vi "_CSM Module Switcher.vi"() -> ()   [LabVIEW 2017]
uses:
  _Support/Typedef/_CSM_GlobalLog_MSG.ctl
  _Support/Typedef/_CSM_Response Source Message.ctl
  _Support/Typedef/_CSM_GlobalLog_MSG_TYPE.ctl
  _Support/Common/Format Timestamp.vi
  AdvanceAPI/CSM - Convert Error to Argument.vi
  <vilib>/Utility/error.llb/Clear Errors.vi
  _Support/GlobalEvent/Gevt-ThreadQueueName.vi
  AdvanceAPI/CSM - Keywords.vi
  _Support/Common/Trim Single line Text.vi
  AdvanceAPI/CSM - Make String Arguments Safe.vi
  _Support/GlobalEvent/FGV-GlobalEventRef.vi
  _Support/FGV-BroadcastRegistry/global-CSMQ FGV Change Flag.vi
  _Support/CSMQ/_CSMOFGV.vi
  Communicable State Machine.lvlib
  _Support/csm-tool-support.lvlib
panel:
  in  "Refresh CSMs Button":bool
  in  "CSM":string(combo)
  in  "Toolbar.Open FP":bool
  in  "Toolbar.Open BD":bool
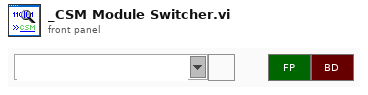
[diagram p1: front panel]
types:
  T1 = typedef "Communicable State Machine.lvlib/_CSM_GlobalLog_MSG.ctl" = cluster{"Name(\"\" to use uuid)":string, "Current State":string, "Arguments":string, "Source Message":T2, "Source Module":string, "Complete(T)/Start(F)":bool, "LogType":T3}
  T2 = typedef "Communicable State Machine.lvlib/_CSM_Response Source Message.ctl" = cluster{"‘State":string, "’Arguments":string, "’Error":errorcluster}
  T3 = typedef "Communicable State Machine.lvlib/_CSM_GlobalLog_MSG_TYPE.ctl" = enum16{"User Log", "State Change", "Status", "Interrupt", "Register", "Unregister", "Error Log", "Module Created", "Module Destroyed"}
  T4 = enum32{"Invalid", "Standard", "Closed", "Hidden", "Minimized", "Maximized"}
  T5 = enum32{"invalid app kind", "Development System", "Run Time System", "Student Edition", "Embedded LabVIEW", "Evaluation", "Custom"}
  T6 = cluster{"Shift":bool, "Ctrl":bool, "Alt":bool, "Cmd":bool, "Opt":bool}
  T7 = cluster{"Core":cluster{"Current VI Reference":refnum<vi>, "Close Panel on Exit?":bool}, "CSM Global Log Event":refnum<user-event>, "lvlps File":path, "Toobar.advance":refnum<vi>[]}
  T8 = cluster{"Current VI Reference":refnum<vi>, "Close Panel on Exit?":bool}
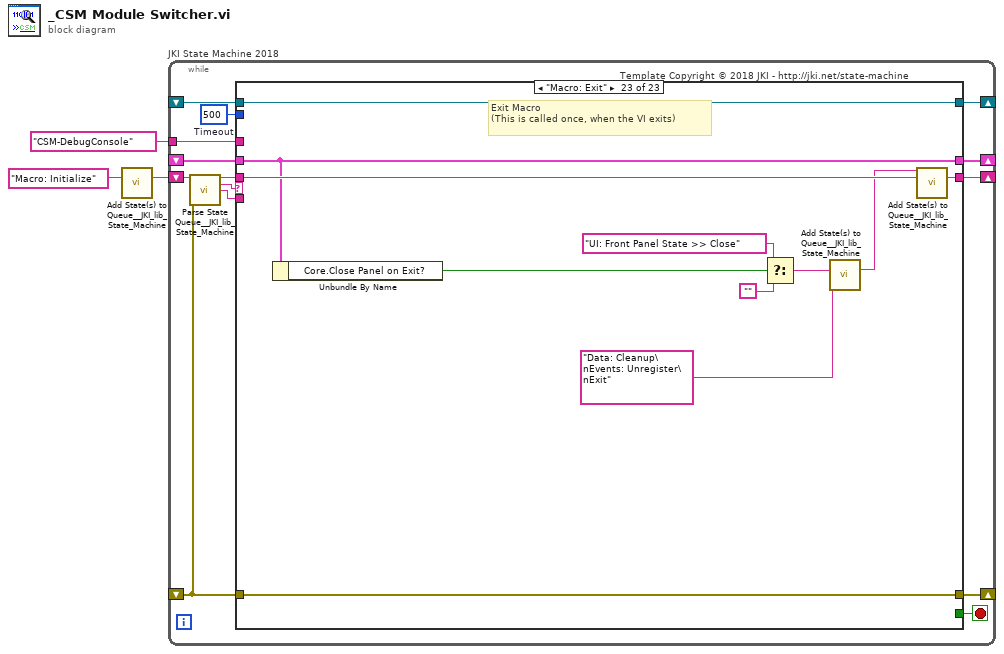
[diagram p0: block diagram]
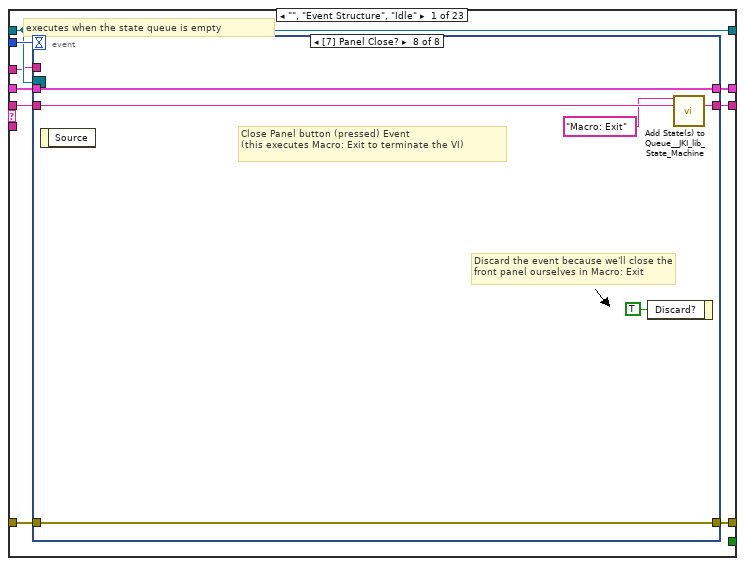
[diagram p2: hidden frame]
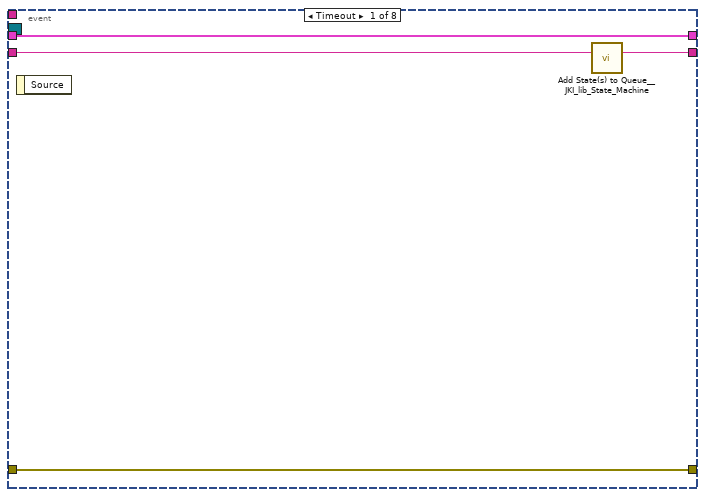
[diagram p3: hidden frame]
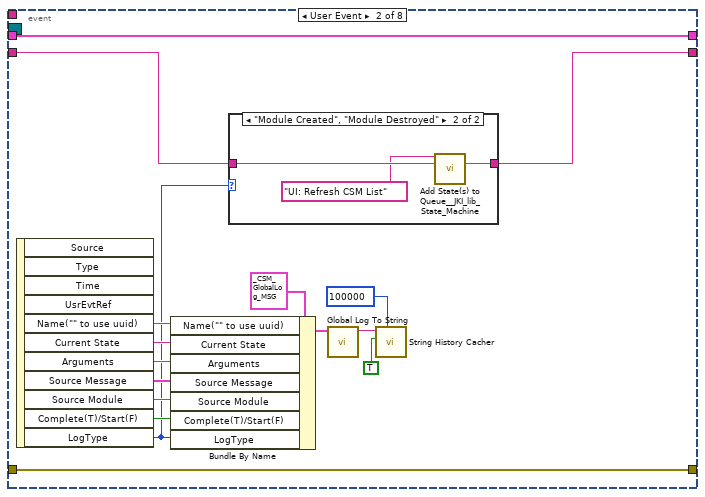
[diagram p4: hidden frame]
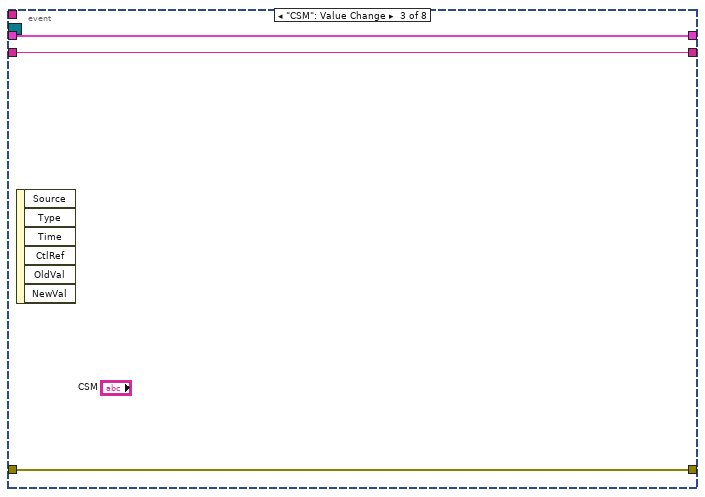
[diagram p6: hidden frame]
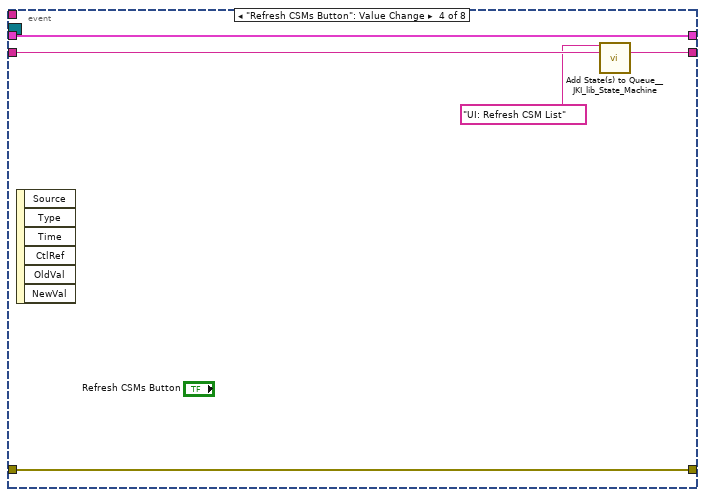
[diagram p7: hidden frame]
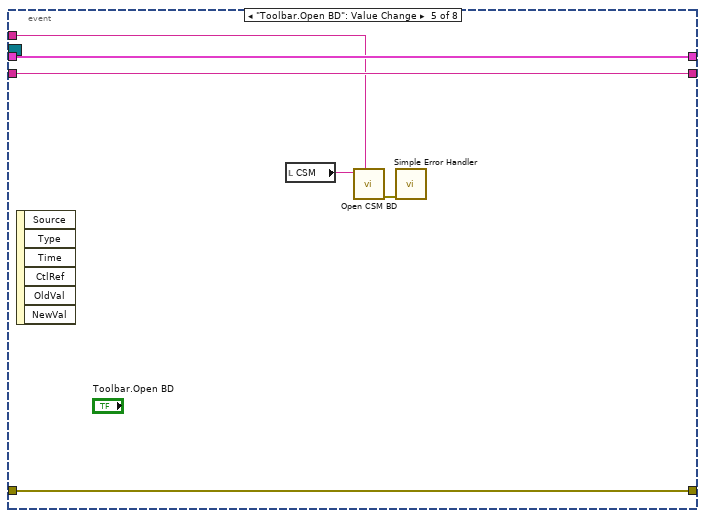
[diagram p8: hidden frame]
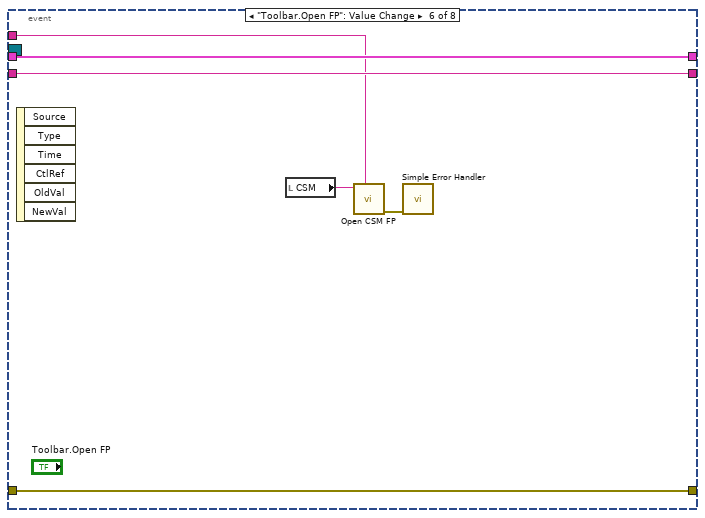
[diagram p9: hidden frame]
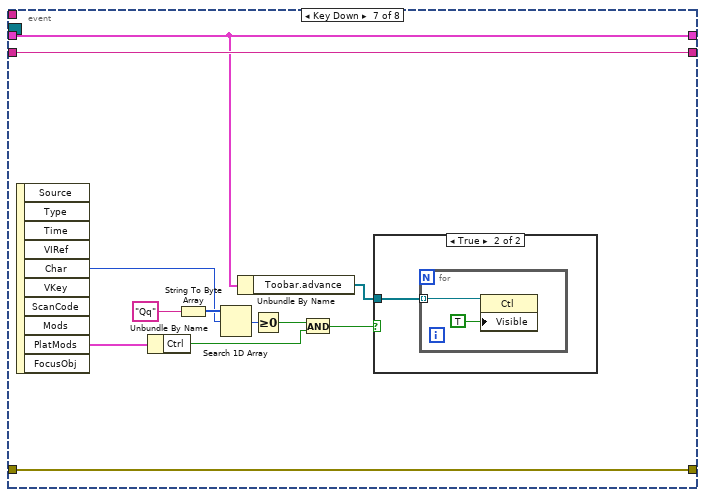
[diagram p10: hidden frame]
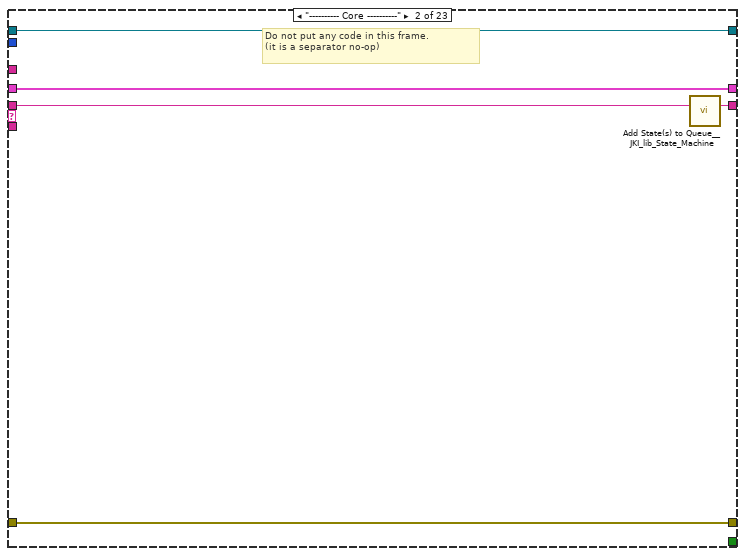
[diagram p12: hidden frame]
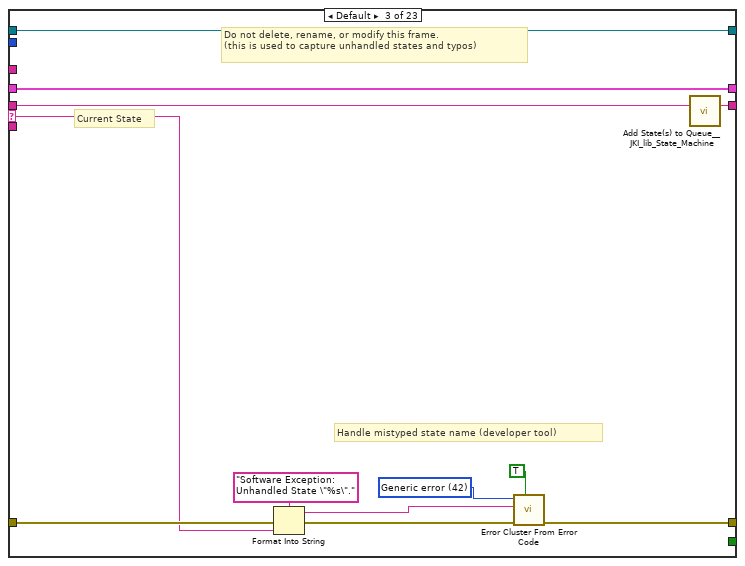
[diagram p13: hidden frame]
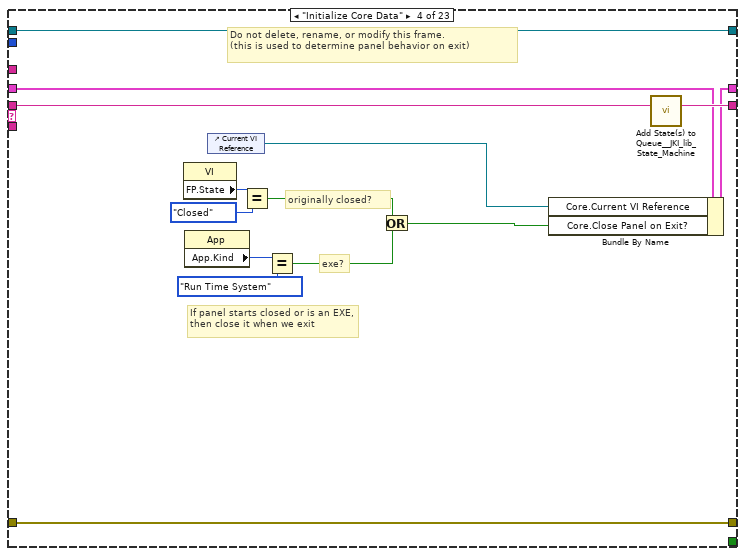
[diagram p14: hidden frame]
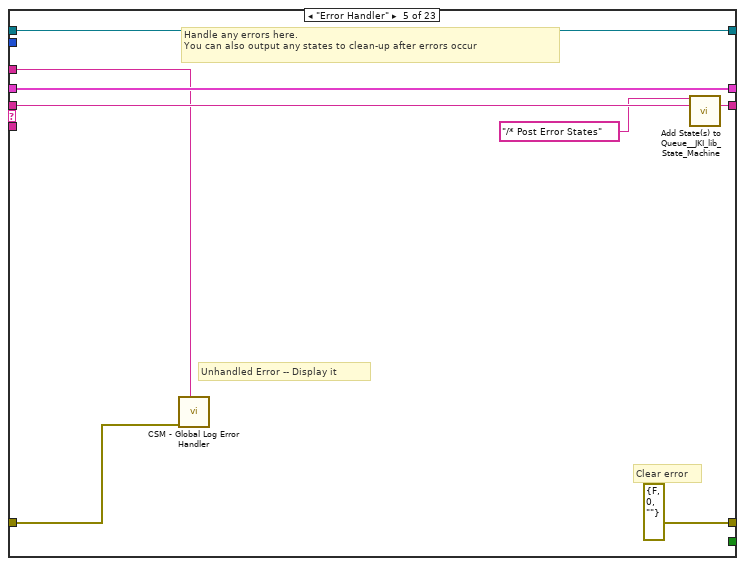
[diagram p15: hidden frame]
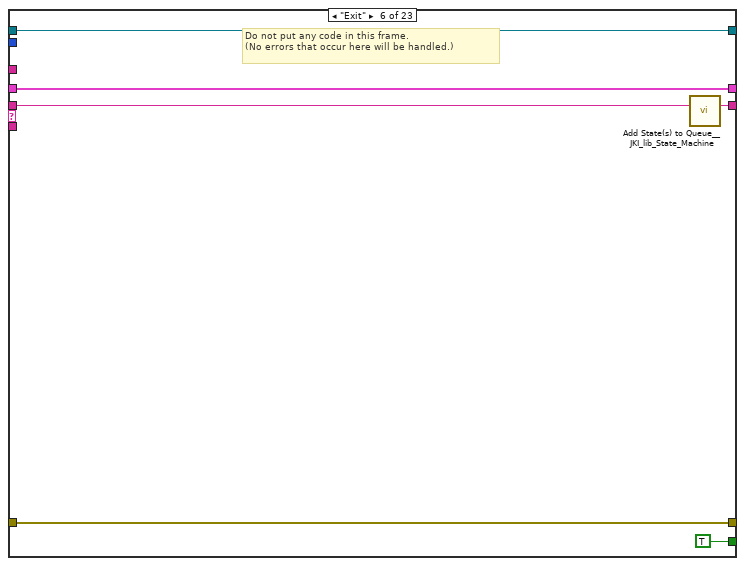
[diagram p16: hidden frame]
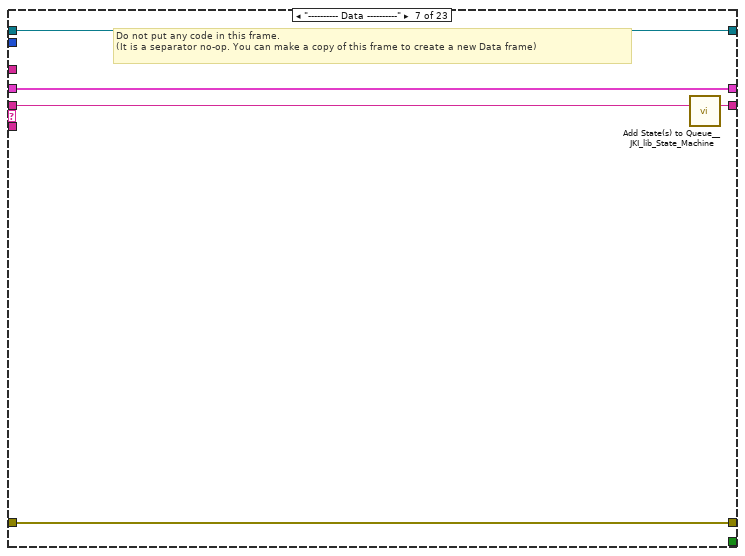
[diagram p17: hidden frame]
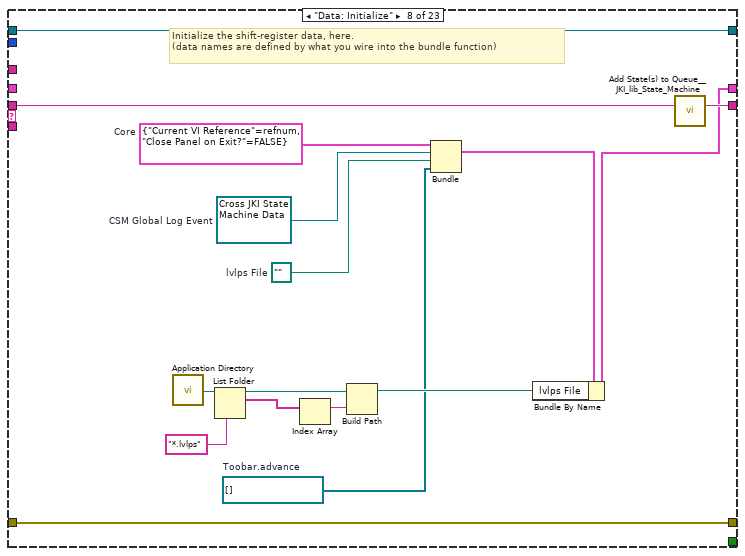
[diagram p18: hidden frame]
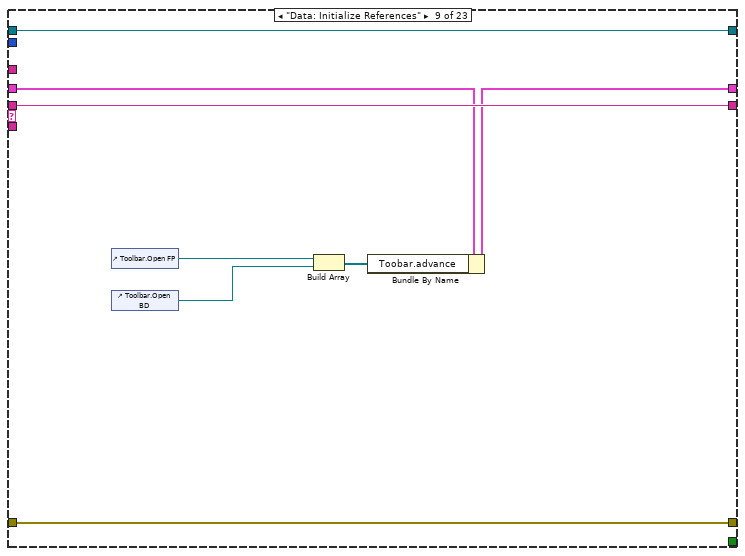
[diagram p19: hidden frame]
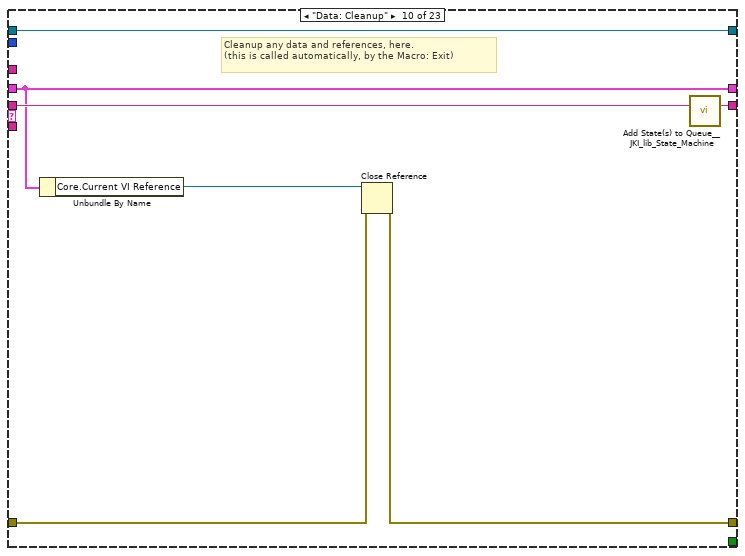
[diagram p20: hidden frame]
diagram:
  n1 = call <vilib>:"Add State(s) to Queue__JKI_lib_State_Machine.vi"("State(s) in (\"\")"="Macro: Initialize") -> ("States Out"=w2:string)  [unwired: 14 in]
  n2 = while "JKI State Machine 2018" {
    shift-right: [w10] -> _
    shift-left: _ -> [w9]
    shift-right: [w13] -> _
    shift-left: _ -> [w7]
    shift-right: [w12] -> _
    shift-left: w2 -> [w14]
    shift-right: [w6] -> _
    shift-left: _ -> [w5]
    tunnel: "CSM-DebugConsole" -> [w4]
    stop <- w11 stop-if-true
    w8 = 500  # Timeout
    # "Template Copyright © 2018 JKI - http://jki.net/state-machine"
    n3 = call <vilib>:"Parse State Queue__JKI_lib_State_Machine.vi"("State Queue"=w14, "Error In (no error)"=w7) -> ("Remaining States"=w16:string, "Current State"=w17:string, "Arguments"=w15:string)  [unwired: 11 in]
    n4 = case shown="\"Macro: Exit\"" w17 {
      selector: w17 -> [_ _ w98 _ _ _ _ _ _ _ _ _ _ _ _ _ _ _ _ _ _ _ _]
      tunnel: w16 -> [w26 w96 w102 w122 w130 w136 w141 w157 w164 w172 w177 w184 w191 w196 w202 w212 w224 w301 w316 w320 w326 w332 w343]
      tunnel: w15 -> [_ _ _ _ _ _ _ _ _ _ _ _ _ _ _ w207 w218 w299 _ _ _ _ _]
      tunnel: w9 -> [w24 w93 w100 w115 w127 w134 w138 _ w163 w167 w174 w182 w187 w193 w198 w210 w220 w296 w315 w318 w323 w329 w340]
      tunnel: [w23 w94 w104 w119 errorcluster {"status"=FALSE, "code"=0, "source"=""} ("error out") w133 w139 w154 w165 w168 w175 w180 w188 w194 w200 w208 w221 w302 w317 w321 w324 w330 w341] -> w13
      tunnel: w7 -> [w22 w94 w103 w119 w126 w133 w139 w154 w165 w169 w175 _ _ w194 w200 w209 w222 w302 w317 w321 w324 w330 w341]
      tunnel: [w25 w95 w101 w121 w129 w135 w140 w156 w164 w171 w176 w183 w190 w195 w201 w211 w223 w301 w316 w320 w325 w331 w342] -> w12
      tunnel: [_ _ _ _ _ TRUE _ _ _ _ _ _ _ _ _ _ _ _ _ _ _ _ _] -> w11
      tunnel: [w21 w93 w100 w120 w127 w134 w138 w149 w159 w167 w174 w182 w187 w193 w198 w210 w220 w296 w315 w318 w323 w329 w340] -> w10
      tunnel: w8 -> [w20 _ _ _ _ _ _ _ _ _ _ _ _ _ _ _ _ _ _ _ _ _ _]
      tunnel: [w19 w92 w97 w109 w124 w131 w137 w152 w162 w166 w173 w181 w189 w192 w199 w206 w217 w300 w314 w319 w322 w327 w333] -> w6
      tunnel: w5 -> [w19 w92 w97 w109 w124 w131 w137 w152 w162 w166 w173 _ w189 w192 w199 w206 w217 w300 w314 w319 w322 w327 w333]
      tunnel: w4 -> [w18 _ _ _ w123 _ _ _ _ _ _ _ _ _ _ _ _ _ _ _ _ _ _]
      frame "", "Event Structure", "Idle" {
        # "executes when the state queue is empty"
        n5 = event shown="[7] Panel Close?" {
          selector: w19 -> [_ _ _ _ _ _ _ _]
          dyn-events: _ -> [_ _ _ _ _ _ _ _]
          timeout: w20 -> [_ _ _ _ _ _ _ _]
          tunnel: w26 -> [w30 w32 w53 w56 w64 w70 w82 w91]
          tunnel: [w29 w33 w53 w55 w64 w70 w82 w90] -> w25
          tunnel: w24 -> [w27 w45 w51 w57 w63 w69 w71 w88]
          tunnel: [w28 w46 w52 w58 w60 w67 w81 w89] -> w23
          tunnel: w22 -> [w28 w46 w52 w58 w60 w67 w81 w89]
          tunnel: [w27 w45 w51 w57 w63 w69 w71 w88] -> w21
          tunnel: w18 -> [_ _ _ _ w59 w65 _ _]
          event Timeout {
            n6 = event-data() -> ()  [unwired: 1 in, 1 out]
            n7 = call <vilib>:"Add State(s) to Queue__JKI_lib_State_Machine.vi"("State(s) in (\"\")"=w30) -> ("States Out"=w29:string)  [unwired: 14 in]
          }
          event User Event {
            n8 = event-data() -> ("Name(\"\" to use uuid)"=w39:string, "Current State"=w38:string, "Arguments"=w37:string, "Source Message"=w36:T2, "Source Module"=w35:string, "Complete(T)/Start(F)"=w34:bool, "LogType"=w31:T3)  [unwired: 1 in, 4 out]
            n9 = Bundle By Name(cluster=T1 {"Name(\"\" to use uuid)"="", "Current State"="", "Arguments"="", "Source Message"={"‘State"="", "’Arguments"="", "’Error"={"status"=FALSE, "code"=0, "source"=""}}, "Source Module"="", "Complete(T)/Start(F)"=FALSE, "LogType"=enum."User Log"} ("Cross CSM Data"), "Name(\"\" to use uuid)"=w39, "Current State"=w38, "Arguments"=w37, "Source Message"=w36, "Source Module"=w35, "Complete(T)/Start(F)"=w34, "LogType"=w31) -> (w44:T1)
            n10 = case shown="\"Module Created\", \"Module Destroyed\"" w31 {
              tunnel: w32 -> [w47 w50]
              tunnel: [w47 w49] -> w33
              frame "User Log", Default {
              }
              frame "Module Created", "Module Destroyed" {
                n11 = call <vilib>:"Add State(s) to Queue__JKI_lib_State_Machine.vi"("State(s) in Front (\"\")"="UI: Refresh CSM List" ("State(s) in Front (\"\")"), "State(s) in (\"\")"=w50) -> ("States Out"=w49:string)  [unwired: 13 in]
              }
            }
            n12 = call "Global Log To String.vi"("Log"=w44) -> ("Log String"=w43:string)  [unwired: 9 in]
            n13 = call "String History Cacher.vi"("length"=100000, "Include Timestamp(T)"=TRUE ("Include Timestamp(F)"), "String"=w43) -> ()  [unwired: 8 in, 1 out]
          }
          event "CSM": Value Change {
            n14 = event-data() -> ()  [unwired: 1 in, 6 out]
          }
          event "Refresh CSMs Button": Value Change {
            n15 = event-data() -> ()  [unwired: 1 in, 6 out]
            n16 = call <vilib>:"Add State(s) to Queue__JKI_lib_State_Machine.vi"("State(s) in Front (\"\")"="UI: Refresh CSM List" ("State(s) in Front (\"\")"), "State(s) in (\"\")"=w56) -> ("States Out"=w55:string)  [unwired: 13 in]
          }
          event "Toolbar.Open BD": Value Change {
            n17 = event-data() -> ()  [unwired: 1 in, 6 out]
            n18 = local read "CSM"() -> (w61:string)
            n19 = call "Open CSM BD.vi"("Current Module(\"\" to generate a ID)"=w59, "CSM"=w61) -> ("error out"=w62:errorcluster)  [unwired: 9 in]
            n20 = call <vilib>:"Simple Error Handler.vi"("error in (no error)"=w62) -> ()  [unwired: 4 in, 5 out]
          }
          event "Toolbar.Open FP": Value Change {
            n21 = event-data() -> ()  [unwired: 1 in, 6 out]
            n22 = local read "CSM"() -> (w68:string)
            n23 = call "Open CSM FP.vi"("Current Module(\"\" to generate a ID)"=w65, "CSM"=w68) -> ("error out"=w66:errorcluster)  [unwired: 9 in]
            n24 = call <vilib>:"Simple Error Handler.vi"("error in (no error)"=w66) -> ()  [unwired: 4 in, 5 out]
          }
          event Key Down {
            n25 = event-data() -> ("Char"=w72:i16, "PlatMods"=w73:T6)  [unwired: 1 in, 8 out]
            n26 = Unbundle By Name(w73) -> ("Ctrl"=w76:bool)
            n27 = String To Byte Array(string="Qq") -> (unsigned byte array=w78:u8[])
            n28 = Search 1D Array(1D array=w78, element=w72) -> (index of element=w79:i32)  [unwired: 1 in]
            n29 = Unbundle By Name(w71) -> ("Toobar.advance"=w74:refnum<vi>[])
            n30 = Greater Or Equal To 0?(x=w79) -> (x >= 0?=w80:bool)
            n31 = And(x=w80, y=w76) -> (x .and. y?=w75:bool)
            n32 = case shown="True" w75 {
              tunnel: w74 -> [_ w83]
              frame False {
              }
              frame True {
                n33 = for {
                  tunnel: w83 -> [w85] mode=indexing
                  n34 = property class="Ctl"(reference=w85, "Visible"=TRUE) -> ()  [unwired: 1 in, 2 out]
                }
              }
            }
          }
          event Panel Close? {
            # "Discard the event because we'll close the front panel ourselves in Macro: Exit"
            # "Close Panel button (pressed) Event\n(this executes Macro: Exit to terminate the VI)"
            n35 = event-data() -> ()  [unwired: 1 in, 1 out]
            n36 = event-data("Discard?"=TRUE) -> ()  [unwired: 1 in, 1 out]
            n37 = call <vilib>:"Add State(s) to Queue__JKI_lib_State_Machine.vi"("State(s) in Front (\"\")"="Macro: Exit", "State(s) in (\"\")"=w91) -> ("States Out"=w90:string)  [unwired: 13 in]
          }
        }
      }
      frame "---------- Core ----------" {
        # "Do not put any code in this frame.\n(it is a separator no-op)"
        n38 = call <vilib>:"Add State(s) to Queue__JKI_lib_State_Machine.vi"("State(s) in (\"\")"=w96) -> ("States Out"=w95:string)  [unwired: 14 in]
      }
      frame Default {
        w107 = 42 items=["No error", "Argument error", "Memory is full", "Out of zone", "End of file", "File already open", "Generic file I/O error", "File not found", "File permission error", "Disk is full", "Duplicate path", "Too many files open", "System feature not enabled", "Resource file not found", "Cannot add resource", "Resource not found", "Image not found", "Image memory error", "Pen does not exist", "Config type invalid", "Config token not found", "Config parse error", "Config memory error", "Bad external code format", "Bad external code offset", "External code not present", "Null window", "Destroy window error", "Null menu", "Print aborted", "Bad print record", "Print driver error", "Windows error during printing", "Memory error during printing", "Print dialog error", "Generic print error", "Invalid device refnum", "Device not found", "Device parameter error", "Device unit error", "Cannot open device", "Device call aborted", "Generic error", "Cancelled by user", "Object ID too low", "Object ID too high", "Object not in heap", "Unknown heap", "Unknown object (invalid DefProc)", "Unknown object (DefProc not in table)", "Message out of range", "Invalid (null) method", "Unknown message", "Manager call not supported", "Bad address", "Network operation in progress", "Network operation timed out", "Connection is busy", "Network attribute not supported", "Network error", "Address in use", "System out of memory", "Connection aborted", "Connection refused", "Not connected", "Already connected", "Connection closed", "Initialization error (interapplication manager)", "Bad occurrence", "Wait on unbound occurrence handler", "Occurrence queue overflow", "Datalog type conflict", "Unused", "Unrecognized type (interapplication manager)", "Memory corrupt", "Failed to make temporary DLL", "Old CIN version", "Drag socket not found", "Failed to load drop-object", "Failed to register OLE object", "Failed to release OLE object", "Format specifier type mismatch", "Unknown format specifier", "Too few format specifiers", "Too many format specifiers", "Scan failed", "Newer CIN version", "Error converting to variant", "Runtime menu error", "Password tampered", "Variant attribute not found", "Incompatible variant data type", "Event data is not available", "Event Store is not present", "Occurrence is not found", "Event Queue is not created", "Event info is not available", "Refnum passed is NULL", "Error retrieving Class GUID", "Error retrieving CoClass GUID", "Error retrieving TypeLib GUID.", "Bad built application magic bytes.", "Specific driver is different from the specific driver associated with the Logical Name.", "There is no session opened to the class driver.", "Max Error", "MAX - Error with config objects", "MAX - Error loading configuration", "MAX - Group not supported"]
        # "Current State"
        # "Do not delete, rename, or modify this frame.\n(this is used to capture unhandled states and typos)"
        # "Handle mistyped state name (developer tool)"
        n39 = Format Into String(format string="Software Exception: Unhandled State \"%s\"." ("message"), error in=w103, w98) -> (resulting string=w106:string, error out=w105:errorcluster)  [unwired: 1 in]
        n40 = call <vilib>:"Error Cluster From Error Code.vi"("show call chain? (False)"=TRUE, "error in (no error)"=w105, "error message (\"\")"=w106, "error code (0)"=w107) -> ("error out"=w104:errorcluster)  [unwired: 5 in]
        n41 = call <vilib>:"Add State(s) to Queue__JKI_lib_State_Machine.vi"("State(s) in (\"\")"=w102) -> ("States Out"=w101:string)  [unwired: 14 in]
      }
      frame "Initialize Core Data" {
        # "Do not delete, rename, or modify this frame.\n(this is used to determine panel behavior on exit)"
        # "originally closed?"
        # "exe?"
        # "If panel starts closed or is an EXE, then close it when we exit"
        n42 = property class="VI"() -> ("FP.State"=w112:T4)  [unwired: 2 in, 2 out]
        n43 = property class="App"() -> ("App.Kind"=w118:T5)  [unwired: 2 in, 2 out]
        n44 = control-ref of="Current VI Reference"() -> (w113:refnum<vi>)
        n45 = Equal?(x=w112, y=T4."Closed" ("Front Panel Window:State")) -> (x = y?=w110:bool)
        n46 = Equal?(x=w118, y=T5."Run Time System" ("Application:Kind")) -> (x = y?=w116:bool)
        n47 = Or(x=w110, y=w116) -> (x .or. y?=w114:bool)
        n48 = Bundle By Name(cluster=w115, "Core.Current VI Reference"=w113, "Core.Close Panel on Exit?"=w114) -> (w120:T7)
        n49 = call <vilib>:"Add State(s) to Queue__JKI_lib_State_Machine.vi"("State(s) in (\"\")"=w122) -> ("States Out"=w121:string)  [unwired: 14 in]
      }
      frame "Error Handler" {
        # "Unhandled Error -- Display it"
        # "Handle any errors here.\nYou can also output any states to clean-up after errors occur"
        # "Clear error"
        n50 = call "CSM - Global Log Error Handler.vi"("Place(\"\" to use VI's Name)"=w123, "Error in"=w126) -> ()  [unwired: 9 in, 1 out]
        n51 = call <vilib>:"Add State(s) to Queue__JKI_lib_State_Machine.vi"("State(s) in Front (\"\")"="/* Post Error States", "State(s) in (\"\")"=w130) -> ("States Out"=w129:string)  [unwired: 13 in]
      }
      frame "Exit" {
        # "Do not put any code in this frame.\n(No errors that occur here will be handled.)"
        n52 = call <vilib>:"Add State(s) to Queue__JKI_lib_State_Machine.vi"("State(s) in (\"\")"=w136) -> ("States Out"=w135:string)  [unwired: 14 in]
      }
      frame "---------- Data ----------" {
        # "Do not put any code in this frame.\n(It is a separator no-op. You can make a copy of this frame to create a new Data frame)"
        n53 = call <vilib>:"Add State(s) to Queue__JKI_lib_State_Machine.vi"("State(s) in (\"\")"=w141) -> ("States Out"=w140:string)  [unwired: 14 in]
      }
      frame "Data: Initialize" {
        w142 = refnum<vi>[] []  # Toobar.advance
        w150 = path ""  # lvlps File
        w151 = refnum<user-event> refnum  # CSM Global Log Event
        w153 = T8 {"Current VI Reference"=refnum, "Close Panel on Exit?"=FALSE}  # Core
        # "Initialize the shift-register data, here.\n(data names are defined by what you wire into the bundle function)"
        n54 = call <vilib>:"Application Directory.vi"() -> ("Application Directory"=w147:path)
        n55 = List Folder(path=w147, pattern="*.lvlps" ("pattern(ini by default)")) -> (path out=w146:path, filenames=w145:string[])  [unwired: 2 in, 2 out]
        n56 = Index Array(array=w145) -> (element=w143:string)  [unwired: 1 in]
        n57 = Build Path(base path=w146, name or relative path=w143) -> (appended path=w144:path)
        n58 = Bundle("Core"=w153, "CSM Global Log Event"=w151, "lvlps File"=w150, "Toobar.advance"=w142) -> (w155:T7)  [unwired: 1 in]
        n59 = Bundle By Name(cluster=w155, "lvlps File"=w144) -> (w149:T7)
        n60 = call <vilib>:"Add State(s) to Queue__JKI_lib_State_Machine.vi"("State(s) in (\"\")"=w157) -> ("States Out"=w156:string)  [unwired: 14 in]
      }
      frame "Data: Initialize References" {
        n61 = control-ref of="Toolbar.Open FP"() -> (w161:refnum<vi>)
        n62 = control-ref of="Toolbar.Open BD"() -> (w160:refnum<vi>)
        n63 = Build Array(w161, w160) -> (w158:refnum<vi>[])
        n64 = Bundle By Name(cluster=w163, "Toobar.advance"=w158) -> (w159:T7)
      }
      frame "Data: Cleanup" {
        # "Cleanup any data and references, here.\n(this is called automatically, by the Macro: Exit)"
        n65 = Unbundle By Name(w167) -> ("Core.Current VI Reference"=w170:refnum<vi>)
        n66 = Close Reference(reference=w170, error in (no error)=w169) -> (error out=w168:errorcluster)
        n67 = call <vilib>:"Add State(s) to Queue__JKI_lib_State_Machine.vi"("State(s) in (\"\")"=w172) -> ("States Out"=w171:string)  [unwired: 14 in]
      }
      frame "---------- Events ----------" {
        # "Do not put any code in this frame.\n(It is a separator no-op. You can make a copy of this frame to create a new UI frame)"
        n68 = call <vilib>:"Add State(s) to Queue__JKI_lib_State_Machine.vi"("State(s) in (\"\")"=w177) -> ("States Out"=w176:string)  [unwired: 14 in]
      }
      frame "Events: Register" {
        # "Do not put any code in this frame.\n(It is a separator no-op. You can make a copy of this frame to create a new UI frame)"
        n69 = call "CSM - Global Log Event.vi"() -> ("Error out"=w178:errorcluster, "CSM Global Log Event"=w179:refnum<user-event>)  [unwired: 10 in]
        n70 = register-events(error in=w178, w179) -> (reference out=w181:refnum<event-registration>, error out=w180:errorcluster)  [unwired: 1 in]
        n71 = call <vilib>:"Add State(s) to Queue__JKI_lib_State_Machine.vi"("State(s) in (\"\")"=w184) -> ("States Out"=w183:string)  [unwired: 14 in]
      }
      frame "Events: Unregister" {
        # "Do not put any code in this frame.\n(It is a separator no-op. You can make a copy of this frame to create a new UI frame)"
        n72 = Unbundle By Name(w187) -> ("CSM Global Log Event"=w186:refnum<user-event>)
        n73 = call "CSM - Destroy Global Log Event.vi"("CSM Global Log Event"=w186) -> ("Error out"=w185:errorcluster)  [unwired: 10 in]
        n74 = Unregister For Events(event registration refnum=w189, error in=w185) -> (error out=w188:errorcluster)
        n75 = call <vilib>:"Add State(s) to Queue__JKI_lib_State_Machine.vi"("State(s) in (\"\")"=w191) -> ("States Out"=w190:string)  [unwired: 14 in]
      }
      frame "---------- UI ----------" {
        # "Do not put any code in this frame.\n(It is a separator no-op. You can make a copy of this frame to create a new UI frame)"
        n76 = call <vilib>:"Add State(s) to Queue__JKI_lib_State_Machine.vi"("State(s) in (\"\")"=w196) -> ("States Out"=w195:string)  [unwired: 14 in]
      }
      frame "UI: Initialize" {
        # "Initialize the User Interface, here.\n(this is called automatically, by the Macro: Init)"
        n77 = Unbundle By Name(w198) -> ("Toobar.advance"=w197:refnum<vi>[])
        n78 = disable-structure shown="Disabled" {
          disable-tunnel: w197 -> [w203 _]
          frame Disabled {
            n79 = for {
              tunnel: w203 -> [w205] mode=indexing
              n80 = property class="Ctl"(reference=w205, "Visible"=FALSE) -> ()  [unwired: 1 in, 2 out]
            }
          }
          frame Enabled {
          }
        }
        n81 = call <vilib>:"Add State(s) to Queue__JKI_lib_State_Machine.vi"("State(s) in (\"\")"=w202) -> ("States Out"=w201:string)  [unwired: 14 in]
      }
      frame "UI: Cursor Set" {
        # "Argument"
        # "Set and Unset Cursor Busy.\n(Usage: \"UI: Cursor Set >> Busy|Idle\")"
        n82 = case shown="\"Idle\", Default" w207 {
          tunnel: w209 -> [w214 w216]
          tunnel: [w213 w215] -> w208
          frame "Idle", Default {
            n83 = call <vilib>:"Unset Busy.vi"("error in (no error)"=w214) -> ("error out"=w213:errorcluster)  [unwired: 10 in]
          }
          frame "Busy" {
            n84 = call <vilib>:"Set Busy.vi"("error in (no error)"=w216) -> ("error out"=w215:errorcluster)  [unwired: 9 in, 1 out]
          }
        }
        n85 = call <vilib>:"Add State(s) to Queue__JKI_lib_State_Machine.vi"("State(s) in (\"\")"=w212) -> ("States Out"=w211:string)  [unwired: 14 in]
      }
      frame "UI: Front Panel State" {
        # "Argument"
        # "Set Front Panel Open or Closed\n(Usage: \"UI: Front Panel State >> Open|Close\")"
        n86 = Unbundle By Name(w220) -> ("Core.Current VI Reference"=w219:refnum<vi>)
        n87 = case shown="\"Minimize\", \"Minimized\"" w218 {
          tunnel: w222 -> [w230 w245 w256 w269 w282]
          tunnel: [w232 w246 w258 w271 w284] -> w221
          tunnel: w219 -> [w231 w243 w257 w270 w283]
          frame "Open", "Standard", Default {
            w225 = T4."Standard" ("State")
            n88 = property class="VI"(reference=w231, error in=w230) -> (reference out=w228:refnum<vi>, error out=w229:errorcluster, "FP.State"=w227:T4)
            n89 = Not Equal?(x=w227, y=w225) -> (x != y?=w226:bool)
            n90 = case shown="True" w226 {
              tunnel: [w236 w238] -> w232
              tunnel: w229 -> [w235 w238]
              tunnel: w228 -> [w234 _]
              tunnel: w225 -> [w233 _]
              frame True {
                n91 = invoke class="VI" method="FP.Open"(reference=w234, error in=w235, "Activate"=TRUE, "State"=w233) -> (error out=w236:errorcluster)  [unwired: 1 in, 4 out]
              }
              frame False {
              }
            }
          }
          frame "Close", "Closed" {
            n92 = property class="VI"(reference=w243, error in=w245) -> (reference out=w242:refnum<vi>, error out=w244:errorcluster, "FP.State"=w240:T4)
            n93 = Not Equal?(x=w240, y=T4."Closed" ("Front Panel Window:State")) -> (x != y?=w239:bool)
            n94 = case shown="True" w239 {
              tunnel: [w247 w250] -> w246
              tunnel: w244 -> [w247 w249]
              tunnel: w242 -> [_ w248]
              frame False {
              }
              frame True {
                n95 = invoke class="VI" method="FP.Close"(reference=w248, error in=w249) -> (error out=w250:errorcluster)  [unwired: 1 in, 2 out]
              }
            }
          }
          frame "Hidden", "Hide" {
            w251 = T4."Hidden" ("State")
            n96 = property class="VI"(reference=w257, error in=w256) -> (reference out=w254:refnum<vi>, error out=w255:errorcluster, "FP.State"=w253:T4)
            n97 = Not Equal?(x=w253, y=w251) -> (x != y?=w252:bool)
            n98 = case shown="True" w252 {
              tunnel: [w262 w263] -> w258
              tunnel: w255 -> [w261 w263]
              tunnel: w254 -> [w260 _]
              tunnel: w251 -> [w259 _]
              frame True {
                n99 = invoke class="VI" method="FP.Open"(reference=w260, error in=w261, "State"=w259) -> (error out=w262:errorcluster)  [unwired: 2 in, 4 out]
              }
              frame False {
              }
            }
          }
          frame "Minimize", "Minimized" {
            w264 = T4."Minimized" ("State")
            n100 = property class="VI"(reference=w270, error in=w269) -> (reference out=w267:refnum<vi>, error out=w268:errorcluster, "FP.State"=w266:T4)
            n101 = Not Equal?(x=w266, y=w264) -> (x != y?=w265:bool)
            n102 = case shown="True" w265 {
              tunnel: [w275 w276] -> w271
              tunnel: w268 -> [w274 w276]
              tunnel: w267 -> [w273 _]
              tunnel: w264 -> [w272 _]
              frame True {
                n103 = invoke class="VI" method="FP.Open"(reference=w273, error in=w274, "State"=w272) -> (error out=w275:errorcluster)  [unwired: 2 in, 4 out]
              }
              frame False {
              }
            }
          }
          frame "Maximize", "Maximized" {
            w277 = T4."Maximized" ("State")
            n104 = property class="VI"(reference=w283, error in=w282) -> (reference out=w280:refnum<vi>, error out=w281:errorcluster, "FP.State"=w279:T4)
            n105 = Not Equal?(x=w279, y=w277) -> (x != y?=w278:bool)
            n106 = case shown="True" w278 {
              tunnel: [w288 w289] -> w284
              tunnel: w281 -> [w287 w289]
              tunnel: w280 -> [w286 _]
              tunnel: w277 -> [w285 _]
              frame True {
                n107 = invoke class="VI" method="FP.Open"(reference=w286, error in=w287, "State"=w285) -> (error out=w288:errorcluster)  [unwired: 2 in, 4 out]
              }
              frame False {
              }
            }
          }
        }
        n108 = call <vilib>:"Add State(s) to Queue__JKI_lib_State_Machine.vi"("State(s) in (\"\")"=w224) -> ("States Out"=w223:string)  [unwired: 14 in]
      }
      frame "UI: Autoset Arguments" {
        n109 = call "CSM - Revert Arguments-Safe String.vi"("Safe Argurment String"=w299) -> ("Origin Argurment String"=w297:string)  [unwired: 8 in]
        n110 = control-ref of="CSM"() -> (w295:refnum<vi>)
        n111 = call "Remove Comments from Line.vi"("single-line text"=w297) -> ("single-line text without comments"=w298:string)  [unwired: 2 in]
        n112 = call "Splite Single-line Message.vi"("single-line text"=w298) -> ("source/target"=w292:string)  [unwired: 6 in, 3 out]
        n113 = property on="Property Node" class="CmbBox"(reference=w295) -> (reference out=w293:refnum<vi>, "Strings[]"=w294:string[])  [unwired: 1 in, 1 out]
        n114 = Search 1D Array(1D array=w294, element=w292) -> (index of element=w291:i32)  [unwired: 1 in]
        n115 = Greater Or Equal To 0?(x=w291) -> (x >= 0?=w290:bool)
        n116 = case shown="False" w290 {
          tunnel: w293 -> [_ w304]
          tunnel: w292 -> [_ w303]
          frame False {
          }
          frame True {
            n117 = property on="Property Node" class="CmbBox"(reference=w304, "Value"=w303) -> ()  [unwired: 1 in, 2 out]
          }
        }
      }
      frame "UI: Refresh CSM List" {
        n118 = control-ref of="CSM"() -> (w313:refnum<vi>)
        n119 = property on="Property Node" class="CmbBox"(reference=w313) -> (reference out=w305:refnum<vi>, "Value"=w309:string)  [unwired: 1 in, 1 out]
        n120 = call "CSM - List Modules.vi"() -> ("Error out"=w312:errorcluster, "Module Names"=w307:string[])  [unwired: 10 in]
        n121 = Search 1D Array(1D array=w307, element=w309) -> (index of element=w311:i32)  [unwired: 1 in]
        n122 = Greater Or Equal To 0?(x=w311) -> (x >= 0?=w310:bool)
        n123 = Index Array(array=w307) -> (element=w308:string)  [unwired: 1 in]
        n124 = Select(t=w309, s=w310, f=w308) -> (s? t:f=w306:string)
        n125 = property on="Property Node" class="CmbBox"(reference=w305, "Strings[]"=w307, "Value"=w306) -> ()  [unwired: 1 in, 2 out]
        n126 = call <vilib>:"Simple Error Handler.vi"("error in (no error)"=w312) -> ()  [unwired: 4 in, 5 out]
      }
      frame "UI: Refresh UI" {
      }
      frame "---------- Macro ----------" {
        # "Do not put any code in this frame.\n(It is a separator no-op. You can make a copy of this frame to create a new Macro frame)"
        n127 = call <vilib>:"Add State(s) to Queue__JKI_lib_State_Machine.vi"("State(s) in (\"\")"=w326) -> ("States Out"=w325:string)  [unwired: 14 in]
      }
      frame "Macro: Initialize" {
        # "Initialization Macro\n(This is called once, when the VI starts)"
        n128 = call <vilib>:"Add State(s) to Queue__JKI_lib_State_Machine.vi"("State(s) in Front (\"\")"="Data: Initialize\nData: Initialize References\nInitialize Core Data\nEvents: Register\nUI: Initialize\nUI: Front Panel State >> Open\nUI: Refresh CSM List\nUI: Refresh UI", "State(s) in (\"\")"=w332) -> ("States Out"=w331:string)  [unwired: 13 in]
      }
      frame "Macro: Exit" {
        # "Exit Macro\n(This is called once, when the VI exits)"
        n129 = Unbundle By Name(w340) -> ("Core.Close Panel on Exit?"=w339:bool)
        n130 = Select(t="UI: Front Panel State >> Close", s=w339, f="") -> (s? t:f=w336:string)
        n131 = call <vilib>:"Add State(s) to Queue__JKI_lib_State_Machine.vi"("State(s) in (\"\")"=w336, "State(s) at Back (\"\")"="Data: Cleanup\nEvents: Unregister\nExit") -> ("States Out"=w334:string)  [unwired: 13 in]
        n132 = call <vilib>:"Add State(s) to Queue__JKI_lib_State_Machine.vi"("State(s) in Front (\"\")"=w334, "State(s) in (\"\")"=w343) -> ("States Out"=w342:string)  [unwired: 13 in]
      }
    }
  }
